vi "Find Turntable Centre.vi"(3 "Mode":T6=enum."Run VI", 5 "Traverse line In":T3={"Start X"=-1250.0, "Start Y"=-250.0, "Start Z"=180.0, "End X"=0.0, "End Y"=0.0, "End Z"=0.0, "No. of pts."=6, "Spacing"=enum."Linear", "Filename"=path "C:/Enflo_Data_Local/2015/EnFlo_Tunnel/Paul_Hayden/Calibrations/Cal_06-2015/Datum_Block_1.xls", "Tunnel Speed"=0.0, "Averaging time (min)"=0.01, "Extra Commands"="", "Carrier_1 Q (l/min)"=nan, "Carrier_2 Q (l/min)"=nan, "Trace Gas Concentration (%)"=nan, "Specific Arguments"="Datum_Image_Calibration.vi  ", "Comments"="", "Row No"=0, "Row Type Selector"=enum."Run VI Named:", "Completion time"="12:51  12-06-2015", "Row Duration (mins)"=0.11291999999999999, "No. of Valid pts."=6, "Meas Setup File"="Trav_Cam_Picture.xls"} {"Carrier_2 Q (l/min)" format="%#.2f"; "Row Duration (mins)" format="%#.1f"; "Row No" min=0; "Trace Gas Concentration (%)" min=0.0 format="%#_4f"; "Carrier_1 Q (l/min)" format="%#.2f"; "Tunnel Speed" format="%#.2f"; "Start X" format="%#.2f"; "Start Y" format="%#.2f"; "Start Z" format="%#.2f"; "End X" format="%#.2f"; "End Y" format="%#.2f"; "End Z" format="%#.2f"; "Averaging time (min)" min=0.0 format="%#.2f"}) -> (0 "Error Message":string, 1 "Status":T2, 2 "Traverse line Out":T3 {"Carrier_2 Q (l/min)" format="%#.2f"; "Row Duration (mins)" format="%#.1f"; "Row No" min=0; "Trace Gas Concentration (%)" min=0.0 format="%#_4f"; "Carrier_1 Q (l/min)" format="%#.2f"; "Tunnel Speed" format="%#.2f"; "Start X" format="%#.2f"; "Start Y" format="%#.2f"; "Start Z" format="%#.2f"; "End X" format="%#.2f"; "End Y" format="%#.2f"; "End Z" format="%#.2f"; "Averaging time (min)" min=0.0 format="%#.2f"})   [LabVIEW 2017]
uses:
  Gen Trav/Traverse_cluster.ctl
  Gen Trav/Spacing.ctl
  Controls/Multi_run_mode.ctl
  Controls/User_Specific_mode.ctl
  Gen Trav/Multi_Run_Status.ctl
  Camera Server/Camera enum/Camera enum.ctl
  Utilities/Image acquisition and processing/Feature detection/Typedefs/Top level controls.ctl
  Utilities/Image acquisition and processing/Feature detection/Typedefs/Theta range.ctl
  Utilities/Image acquisition and processing/Feature detection/Typedefs/Txy range.ctl
  Utilities/Image acquisition and processing/Feature detection/Typedefs/ROI bounds.ctl
  Camera Server/Camera enum/Camera resolution.ctl
  Controls/Setup.ctl
  Controls/Save_Data.ctl
  Globals/Constants_global.vi
  Globals/Dynamic_call_global.ph.vi
panel:
  out "Y Offset":dbl=-999.0 format="%.2f"
  out "X Offset":dbl=-999.0 format="%.2f"
  in  "Camera":T1="Travcam"
  out "Local Log File":path
  out "y radius":dbl
  out "x radius":dbl
  out "y centre 2":dbl
  out "x centre 2":dbl
  in  "stop":bool
  out "radius":dbl
  out "y centre":dbl
  out "x centre":dbl
  out "Y":dbl[](array[numeric])
  out "X":dbl[](array[numeric])
  in  "Radius":dbl=900.0
  # "Circle"
  # "Ellipse"
  # "X           Y            Z"
  # "Start"
  # "End"
  # "X           Y            Z"
  # "Start"
  # "End"
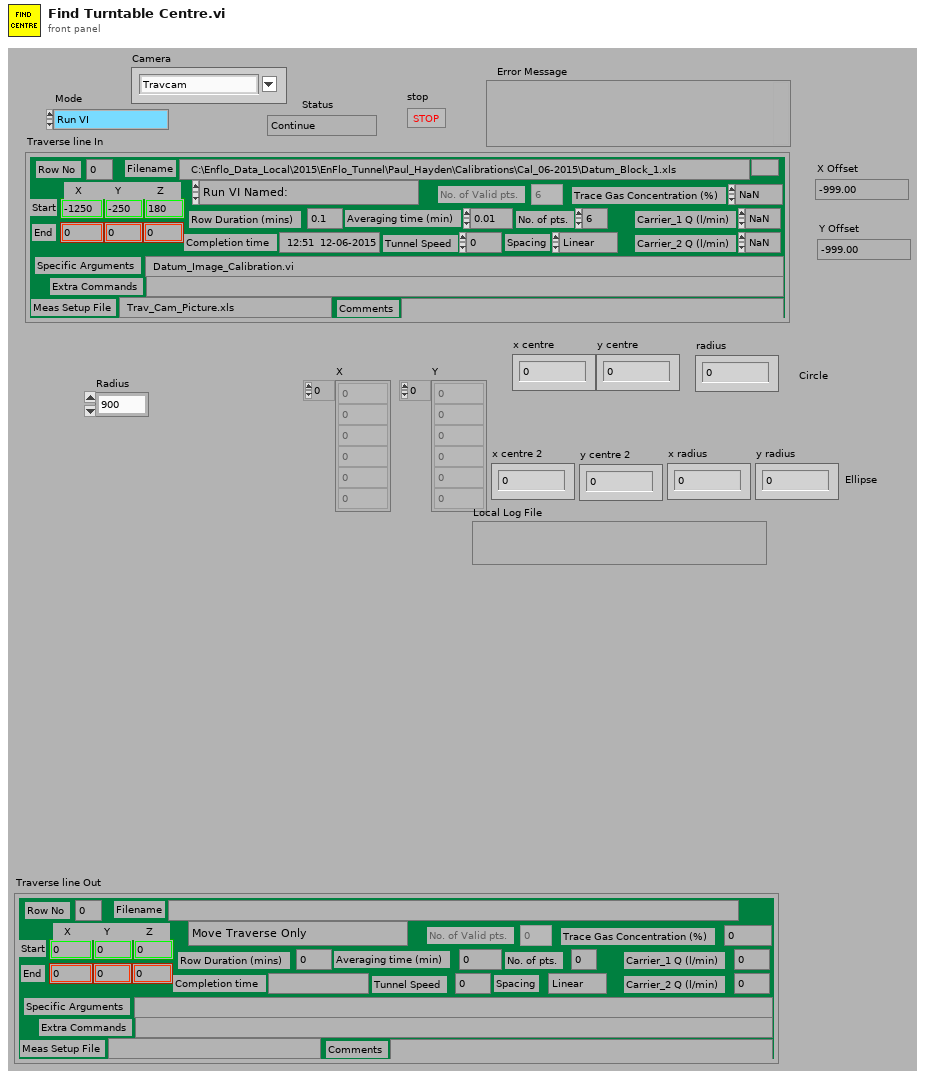
[diagram p1: front panel]
types:
  T1 = typedef "Camera enum.ctl" = string
  T2 = typedef "Multi_Run_Status.ctl" = enum16{"Continue", "Continue with Error", "Jump to Next Point", "Jump to Next Row", "Jump To Fall Back", "Terminate Run"}
  T3 = typedef "Traverse_cluster.ctl" = cluster{"Start X":sgl, "Start Y":sgl, "Start Z":sgl, "End X":sgl, "End Y":sgl, "End Z":sgl, "No. of pts.":i32, "Spacing":T4, "Filename":path, "Tunnel Speed":dbl, "Averaging time (min)":dbl, "Extra Commands":string, "Carrier_1 Q (l/min)":dbl, "Carrier_2 Q (l/min)":dbl, "Trace Gas Concentration (%)":dbl, "Specific Arguments":string, "Comments":string, "Row No":i32, "Row Type Selector":T5, "Completion time":string, "Row Duration (mins)":dbl, "No. of Valid pts.":i32, "Meas Setup File":string}
  T4 = typedef "Spacing.ctl" = enum16{"Linear", "Log", "Gauss", "Specified", "N/A"}
  T5 = typedef "Multi_run_mode.ctl" = enum16{"Move Traverse Only", "Set Tunnel Speed Only", "Set Source Only", "Set Measurement Conditions", "Single Measurement", "Vertical Profile", "Lateral Profile", "Longitudinal Profile", "Explore Volume", "Multi-Axis Profile", "Auto Calibrate", "Meas Fast FID Bkgnd", "Check Beam Power", "Scanning Valve Measurement", "Run VI Named:", "Set ADAM Ch", "Wait (minutes)", "Send Message", "Synchronize With:", "Fall Back to this Row", "Turn Off Row Repeating", "Traverse 3D Volume", "Blank Row", "Jump to Fall Back Row"}
  T6 = typedef "User_Specific_mode.ctl" = enum16{"Check VI only", "Run VI"}
  T7 = typedef "ROI bounds.ctl" = cluster{"Xmax":i32, "Ymax":i32, "Xmin":i32, "Ymin":i32}
  T8 = typedef "Txy range.ctl" = cluster{"Tx max (pix)":i32, "Tx min (pix)":i32, "Ty max (pix)":i32, "Ty min (pix)":i32}
  T9 = typedef "Theta range.ctl" = cluster{"theta max (deg)":dbl, "theta min (deg)":dbl}
  T10 = typedef "Top level controls.ctl" = cluster{"Auto ROI (for rot.)":bool, "Apply scaling":bool, "Apply rotation":bool, "Apply Tx":bool, "Apply Ty":bool, "Keep proc. img":bool}
  T11 = typedef "Save_Data.ctl" = enum16{"Save No Data", "Save Data"}
  T12 = typedef "Setup.ctl" = enum16{"Run Program", "Show Setup", "Save Current Setup", "Setup Front Panel"}
  T13 = typedef "Camera resolution.ctl" = u8
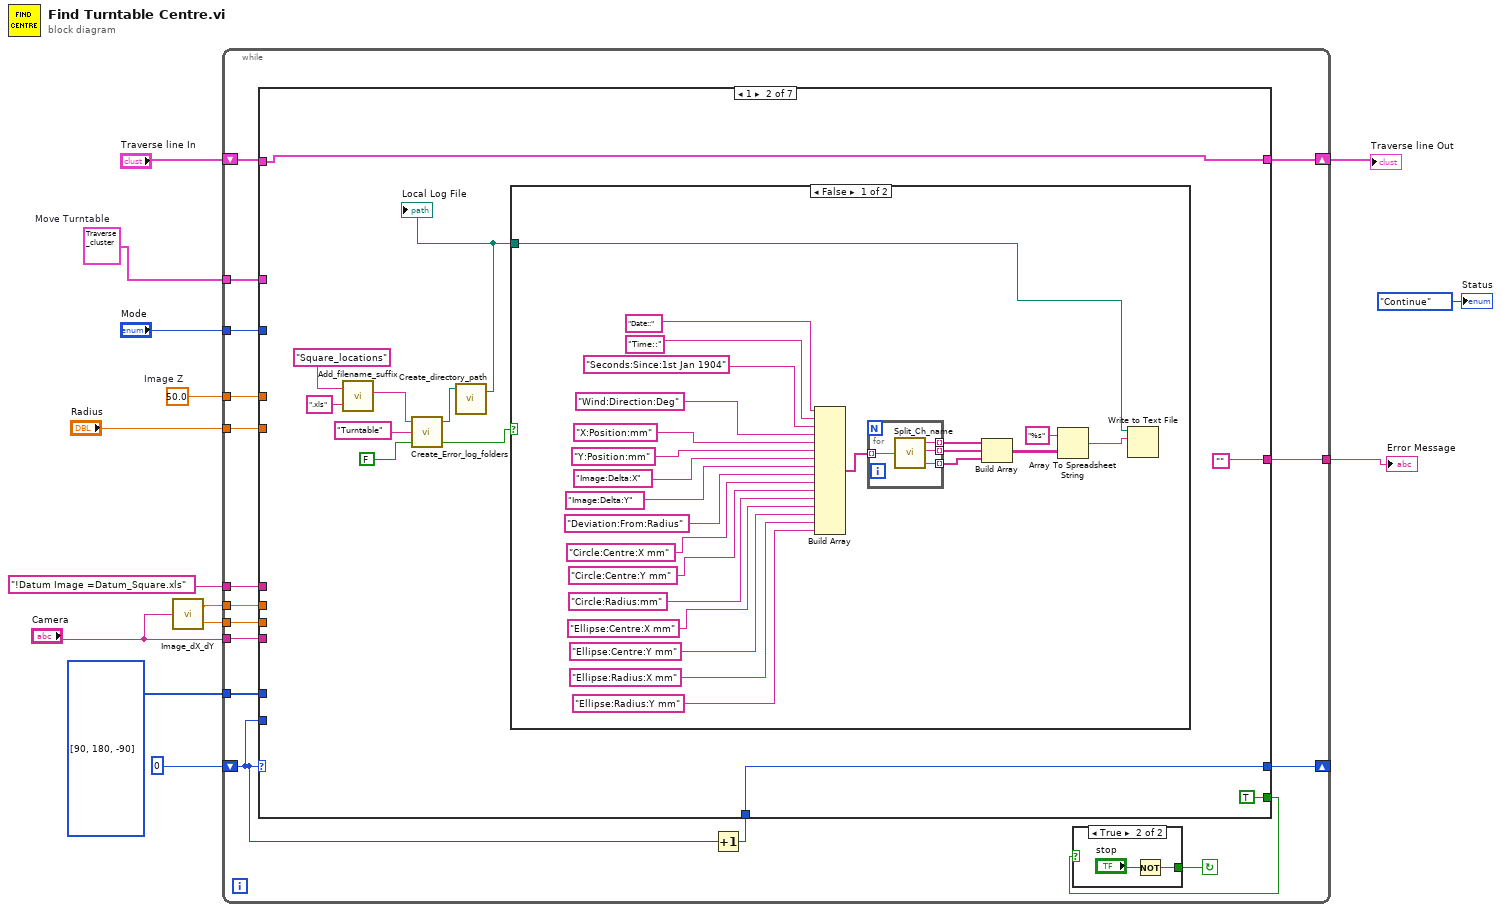
[diagram p0: block diagram]
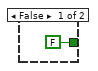
[diagram p2: hidden frame]
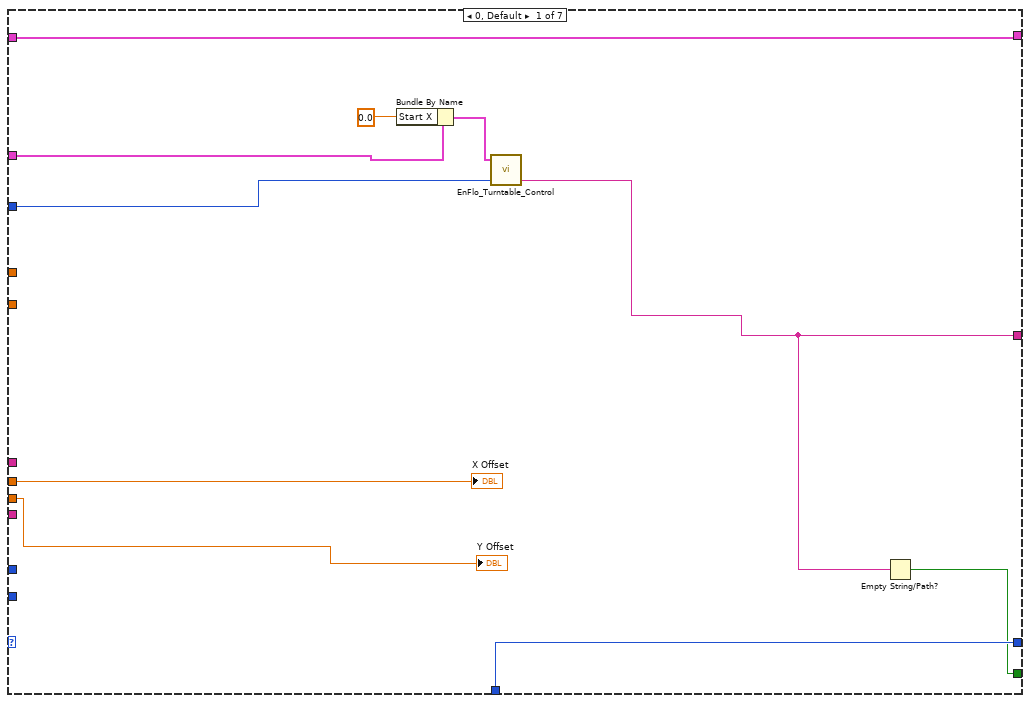
[diagram p3: hidden frame]
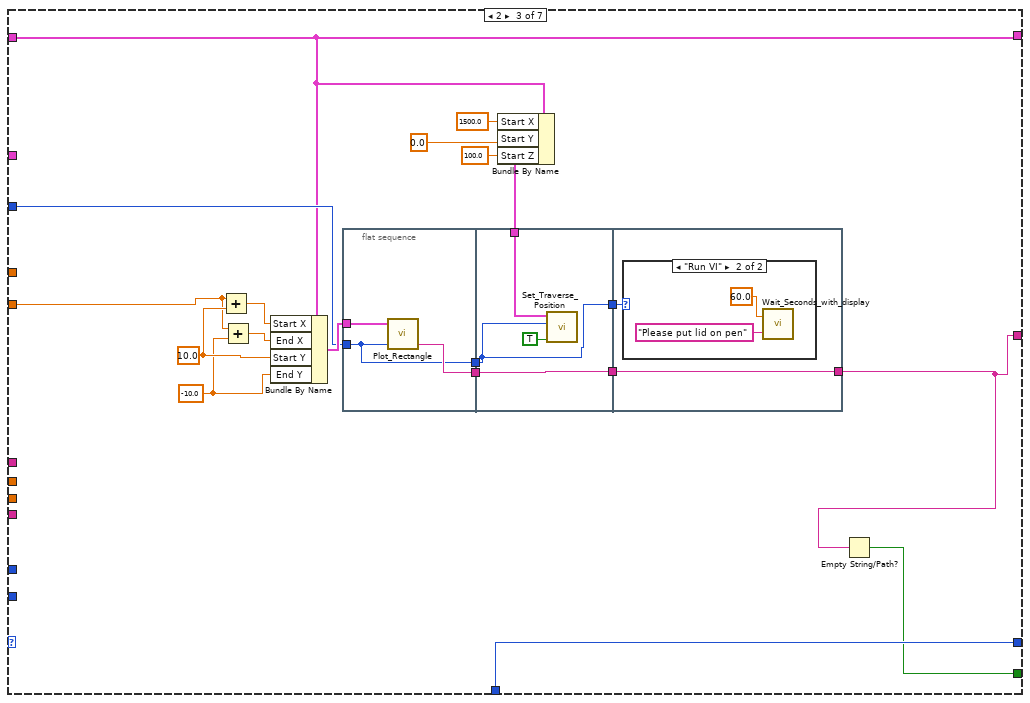
[diagram p5: hidden frame]
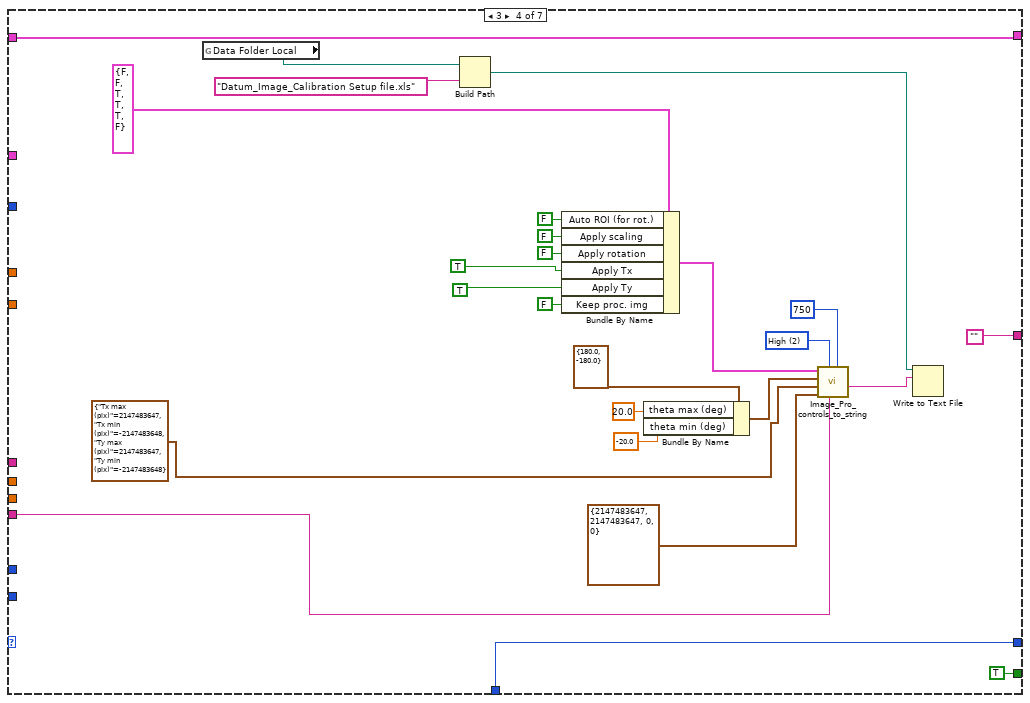
[diagram p7: hidden frame]
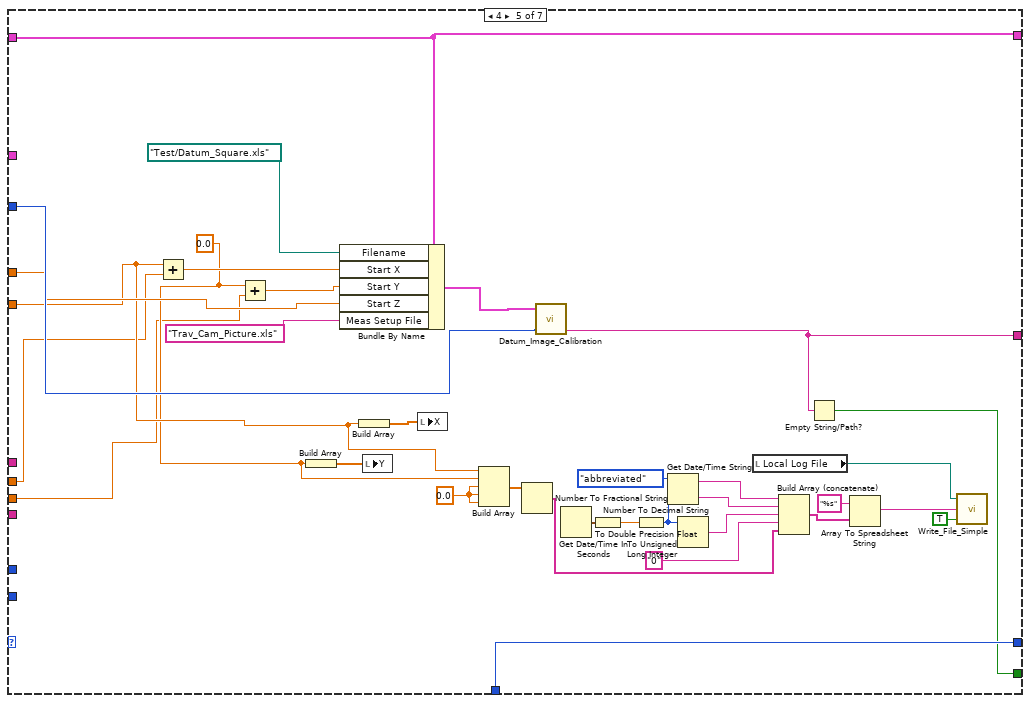
[diagram p8: hidden frame]
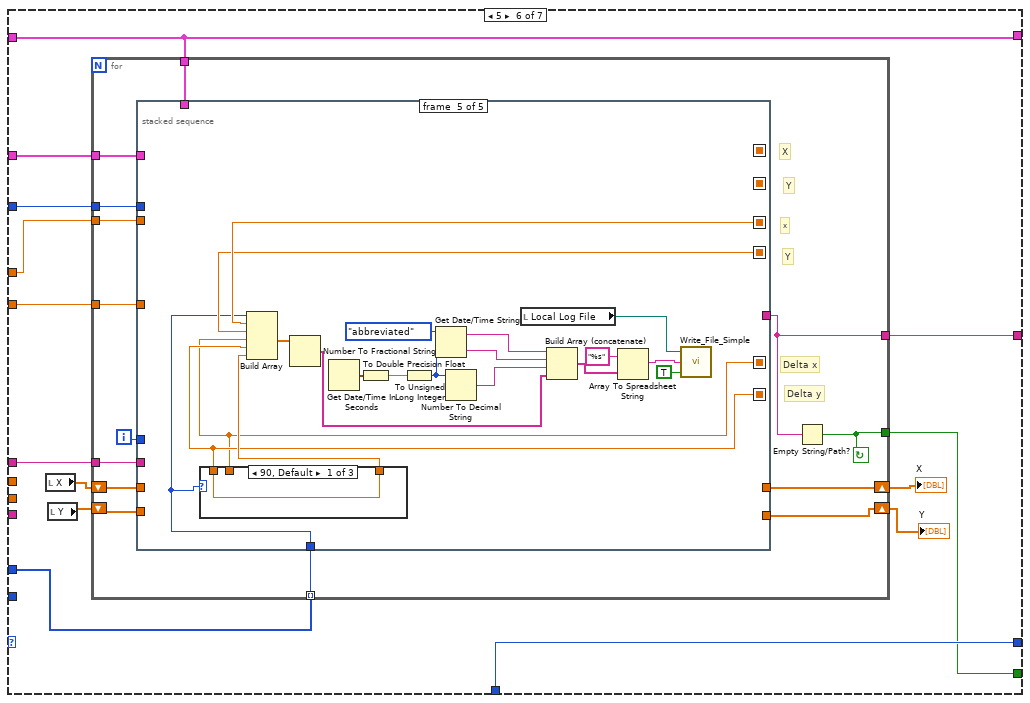
[diagram p9: hidden frame]
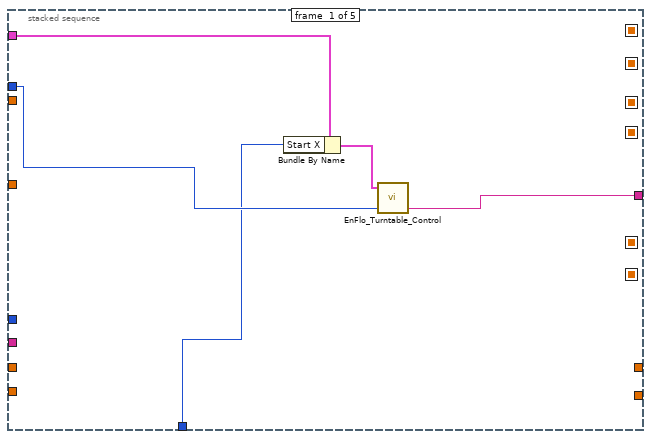
[diagram p10: hidden frame]
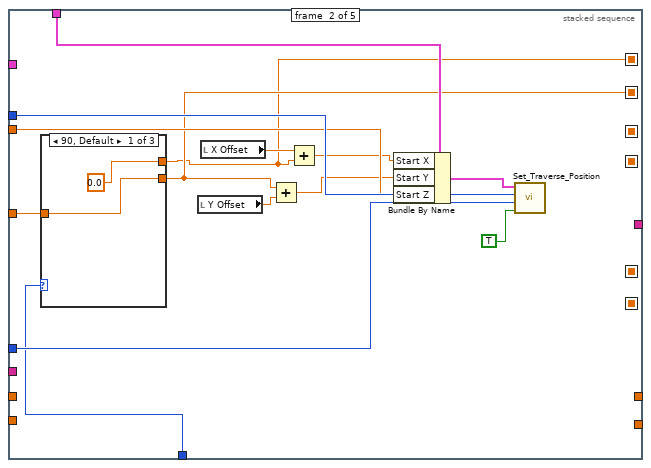
[diagram p11: hidden frame]
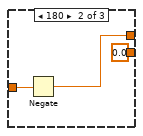
[diagram p12: hidden frame]
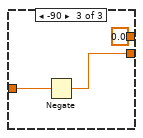
[diagram p13: hidden frame]
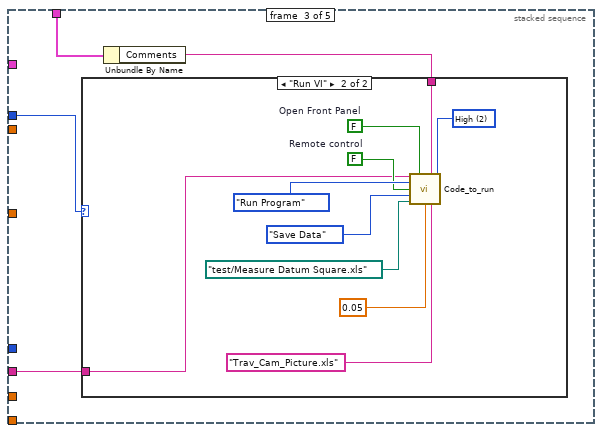
[diagram p14: hidden frame]
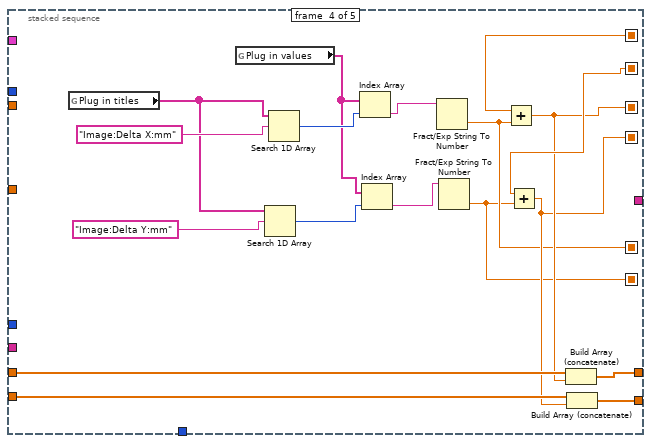
[diagram p16: hidden frame]
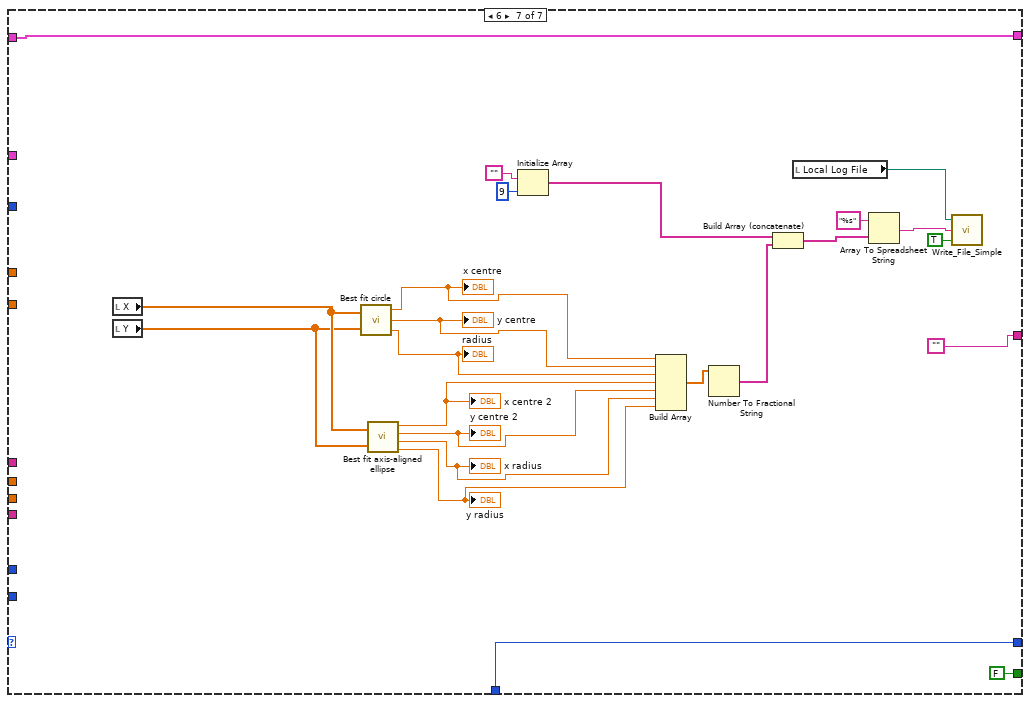
[diagram p19: hidden frame]
diagram:
  w4 = T3 {"Start X"=0.0, "Start Y"=nan, "Start Z"=nan, "End X"=nan, "End Y"=nan, "End Z"=nan, "No. of pts."=0, "Spacing"=enum."N/A", "Filename"=path "  ---------", "Tunnel Speed"=nan, "Averaging time (min)"=nan, "Extra Commands"="!Datum Image = Datum_Turntable.xls", "Carrier_1 Q (l/min)"=nan, "Carrier_2 Q (l/min)"=nan, "Trace Gas Concentration (%)"=nan, "Specific Arguments"="EnFlo_Turntable_Control.vi", "Comments"="", "Row No"=0, "Row Type Selector"=enum."Run VI Named:", "Completion time"="18:36  07-04-2016", "Row Duration (mins)"=0.6666666666666666, "No. of Valid pts."=0, "Meas Setup File"="Trav_Cam_Picture.xls"}  # Move Turntable
  w7 = sgl 50.0  # Image Z
  n1 = call "Image_dX_dY.vi"("Camera"="Camera") -> ("X Offset"=w2:dbl, "Y Offset"=w1:dbl)
  n2 = while {
    shift-left: 0 -> [w27]
    shift-right: [w31] -> _
    tunnel: "Mode" -> [w30]
    shift-right: [w28] -> w11
    shift-left: "Traverse line In" -> [w29]
    tunnel: "Radius" -> [w25]
    tunnel: [w24] -> w9
    tunnel: w7 -> [w23]
    tunnel: i32[] [90, 180, -90] ("appended array") -> [w20]
    tunnel: "!Datum Image =Datum_Square.xls" ("Extra Commands") -> [w19]
    tunnel: w4 -> [w18]
    tunnel: "Camera" -> [w17]
    tunnel: w2 -> [w16]
    tunnel: w1 -> [w15]
    stop <- w21 continue-if-true
    n3 = Increment(x=w27) -> (x+1=w26:i32)
    n4 = case shown="1" w27 {
      tunnel: [w42 TRUE w100 TRUE w168 w183 FALSE] -> w22
      tunnel: [w44 w49 w102 w139 w171 w186 w302] -> w31
      tunnel: w27 -> [_ _ _ _ _ _ _]
      tunnel: w30 -> [w41 _ w101 _ w166 w185 _]
      tunnel: w29 -> [w43 w50 w93 w138 w172 w181 w303]
      tunnel: [w43 w50 w93 w138 w172 w181 w303] -> w28
      tunnel: w26 -> [w44 w49 w102 w139 w171 w186 w302]
      tunnel: w25 -> [_ _ w96 _ w147 w182 _]
      tunnel: [w38 "" w86 "" w165 w184 ""] -> w24
      tunnel: w23 -> [_ _ _ _ w162 w176 _]
      tunnel: w20 -> [_ _ _ _ _ w175 _]
      tunnel: w19 -> [_ _ _ _ _ w174 _]
      tunnel: w18 -> [w37 _ _ _ _ w173 _]
      tunnel: w17 -> [_ _ _ w117 _ _ _]
      tunnel: w16 -> [w36 _ _ _ w144 _ _]
      tunnel: w15 -> [w35 _ _ _ w143 _ _]
      frame 0, Default {
        n5 = Bundle By Name(cluster=w37, "Start X"=sgl 0.0 ("element")) -> (w40:T3)
        n6 = call "EnFlo_Turntable_Control.vi"("Mode"=w41, "Traverse line In"=w40) -> ("Error Message"=w38:string)  [unwired: 1 in, 2 out]
        n7 = Empty String/Path?(string/path=w38) -> (empty?=w42:bool)
        "X Offset" <- w36
        "Y Offset" <- w35
      }
      frame 1 {
        n8 = call "Add_filename_suffix.vi"("Filename"="Square_locations", "Suffix to add"=".xls") -> ("Filename out"=w54:string)  [unwired: 3 out]
        n9 = call "Create_Error_log_folders.vi"("Log Filename"=w54, "Log Folder"="Turntable" ("Input Element"), "Per Day Log File?"=FALSE) -> ("Local Log File"=w46:path, "exists?"=w52:bool)  [unwired: 2 in, 1 out]
        n10 = call "Create_directory_path.vi"("Path name"=w46) -> ("Path name Out"=w45:path)  [unwired: 2 in, 1 out]
        "Local Log File" <- w45
        n11 = case shown="False" w52 {
          tunnel: w45 -> [w67 _]
          frame False {
            n12 = Build Array("Date::", "Time::", "Seconds:Since:1st Jan 1904", "Wind:Direction:Deg", "X:Position:mm", "Y:Position:mm", "Image:Delta:X", "Image:Delta:Y", "Deviation:From:Radius", "Circle:Centre:X mm", "Circle:Centre:Y mm", "Circle:Radius:mm", "Ellipse:Centre:X mm", "Ellipse:Centre:Y mm", "Ellipse:Radius:X mm", "Ellipse:Radius:Y mm") -> (w76:string[])
            n13 = for {
              tunnel: w76 -> [w84] mode=indexing
              tunnel: [w83] -> w75 mode=indexing
              tunnel: [w82] -> w74 mode=indexing
              tunnel: [w81] -> w73 mode=indexing
              n14 = call "Split_Ch_name.vi"("Ch name"=w84) -> ("Top level"=w83:string, "Middle"=w82:string, "Low level"=w81:string)
            }
            n15 = Build Array(w75, w74, w73) -> (w65:string[][])
            n16 = Array To Spreadsheet String(array=w65, 3:"%s" ("format string")) -> (spreadsheet string=w64:string)  [unwired: 1 out]
            n17 = Write to Text File(file (use dialog)=w67, text=w64) -> ()  [unwired: 2 in, 3 out]
          }
          frame True {
          }
        }
      }
      frame 2 {
        w97 = sgl -10.0 ("End Y")
        w98 = sgl 10.0 ("Start Y")
        n18 = Add(x=w96, y=w98) -> (x+y=w99:dbl)
        n19 = Add(x=w96, y=w97) -> (x+y=w95:dbl)
        n20 = Bundle By Name(cluster=w93, "Start X"=w99, "End X"=w95, "Start Y"=w98, "End Y"=w97) -> (w103:T3)
        n21 = flat-sequence {
          tunnel: [w105] -> w94
          tunnel: [w104] -> w88
          tunnel: w103 -> [w106]
          tunnel: w101 -> [w104]
          tunnel: w94 -> [w110]
          tunnel: w89 -> [w109]
          tunnel: w88 -> [w107]
          tunnel: [w110] -> w87
          tunnel: [w107] -> w85
          tunnel: [w112] -> w86
          tunnel: w87 -> [w112]
          tunnel: w85 -> [w111]
          frame #0 {
            n22 = call "Plot_Rectangle.vi"("Mode"=w104, "Traverse line In"=w106) -> ("Error Message"=w105:string)  [unwired: 1 in, 2 out]
          }
          frame #1 {
            n23 = call "Set_Traverse_Position.vi"("Last Part of Move?"=TRUE, "Simulate/Run"=w107, "Traverse line"=w109) -> ()  [unwired: 3 in, 1 out]
          }
          frame #2 {
            n24 = case shown="\"Run VI\"" w111 {
              frame "Check VI only" {
              }
              frame "Run VI" {
                n25 = call "Wait_Seconds_with_display.vi"("Message"="Please put lid on pen", "Seconds to wait"=60.0) -> ()  [unwired: 1 in, 1 out]
              }
            }
          }
        }
        n26 = Bundle By Name(cluster=w93, "Start X"=sgl 1500.0, "Start Y"=sgl 0.0, "Start Z"=sgl 100.0) -> (w89:T3)
        n27 = Empty String/Path?(string/path=w86) -> (empty?=w100:bool)
      }
      frame 3 {
        w116 = T13 2 items=["Low", "Med.", "High", "Max."] ("Resolution")
        n28 = global read "Constants_global.vi" "Data Folder Local"() -> (w136:path)
        n29 = Build Path(base path=w136, name or relative path="Datum_Image_Calibration Setup file.xls") -> (appended path=w121:path)
        n30 = Bundle By Name(cluster=T10 {"Auto ROI (for rot.)"=FALSE, "Apply scaling"=FALSE, "Apply rotation"=TRUE, "Apply Tx"=TRUE, "Apply Ty"=TRUE, "Keep proc. img"=FALSE} ("Controls"), "Auto ROI (for rot.)"=FALSE, "Apply scaling"=FALSE, "Apply rotation"=FALSE, "Apply Tx"=TRUE, "Apply Ty"=TRUE, "Keep proc. img"=FALSE) -> (w128:T10)
        n31 = Bundle By Name(cluster=T9 {"theta max (deg)"=180.0, "theta min (deg)"=-180.0} ("Theta range (deg)"), "theta max (deg)"=20.0, "theta min (deg)"=-20.0) -> (w126:T9)
        n32 = call "Image_Pro_controls_to_string.vi"("Quality"=u32 750, "Camera"=w117, "Resolution"=w116, "ROI to crop (pixels)"=T7 {"Xmax"=2147483647, "Ymax"=2147483647, "Xmin"=0, "Ymin"=0}, "Txy range (pixels)"=T8 {"Tx max (pix)"=2147483647, "Tx min (pix)"=-2147483648, "Ty max (pix)"=2147483647, "Ty min (pix)"=-2147483648}, "Theta range (deg)"=w126, "Controls"=w128) -> ("Setup String"=w122:string)  [unwired: 4 in]
        n33 = Write to Text File(file (use dialog)=w121, text=w122) -> ()  [unwired: 2 in, 3 out]
      }
      frame 4 {
        w152 = 0.0 ("element")
        w146 = sgl 0.0 ("Start Y")
        n34 = Add(x=w147, y=w144) -> (x+y=w153:dbl)
        n35 = Add(x=w146, y=w143) -> (x+y=w145:dbl)
        n36 = Build Array(w146) -> (w163:sgl[])
        n37 = Bundle By Name(cluster=w172, "Filename"=path "Test/Datum_Square.xls", "Start X"=w153, "Start Y"=w145, "Start Z"=w162, "Meas Setup File"="Trav_Cam_Picture.xls") -> (w167:T3)
        n38 = Build Array(w147) -> (w164:dbl[])
        n39 = local write "Y"(w163) -> ()
        n40 = local write "X"(w164) -> ()
        n41 = Build Array(w147, w146, w152, w152, w152) -> (w151:dbl[])
        n42 = Number To Fractional String(number=w151) -> (F-format string=w150:string[])  [unwired: 3 in]
        n43 = call "Datum_Image_Calibration.vi"("Mode"=w166, "Traverse line In"=w167) -> ("Error Message"=w165:string)  [unwired: 1 in, 2 out]
        n44 = Get Date/Time In Seconds() -> (seconds since 1Jan1904=w158:timestamp)
        n45 = To Double Precision Float(number=w158) -> (double precision float=w160:dbl)
        n46 = To Unsigned Long Integer(number=w160) -> (unsigned 32bit integer=w159:u32)
        n47 = Get Date/Time String(date format (0)=enum16{"short", "long", "abbreviated"}."abbreviated", seconds (now)=w159) -> (date string=w157:string, time string=w156:string)  [unwired: 1 out]
        n48 = Number To Decimal String(number=w159) -> (decimal integer string=w155:string)  [unwired: 1 out]
        n49 = local read "Local Log File"() -> (w142:path)
        n50 = Build Array (concatenate)(w157, w156, w155, "0", w150) -> (w148:string[])
        n51 = Empty String/Path?(string/path=w165) -> (empty?=w168:bool)
        n52 = Array To Spreadsheet String(array=w148, 3:"%s" ("format string")) -> (spreadsheet string=w141:string)  [unwired: 1 out]
        n53 = call "Write_File_Simple.vi"("append to file? (new file:F)"=TRUE, "character string"=w141, "file path"=w142) -> ()  [unwired: 2 out]
      }
      frame 5 {
        n54 = local read "X"() -> (w180:dbl[])
        n55 = local read "Y"() -> (w179:dbl[])
        n56 = for {
          tunnel: w185 -> [w200]
          tunnel: [w199] -> w184
          tunnel: [w198] -> w183
          tunnel: w175 -> [w197] mode=indexing
          tunnel: w182 -> [w196]
          tunnel: w181 -> [w195]
          shift-right: [w191] -> w178
          shift-left: w180 -> [w193]
          shift-right: [w190] -> w177
          shift-left: w179 -> [w192]
          tunnel: w176 -> [w189]
          tunnel: w174 -> [w188]
          tunnel: w173 -> [w187]
          i -> [w194]
          stop <- w198 continue-if-true
          # "Y"
          # "X"
          # "Delta y"
          # "Delta x"
          # "Y"
          # "x"
          n57 = stacked-sequence {
            seq-local: [_ w206 _ _ _] -> [_ _ _ w251 _]
            seq-local: [_ w209 _ _ _] -> [_ _ _ w250 _]
            seq-local: [_ _ _ w245 _] -> [_ _ _ _ w268]
            seq-local: [_ _ _ w244 _] -> [_ _ _ _ w267]
            seq-local: [_ _ _ w243 _] -> [_ _ _ _ w263]
            seq-local: [_ _ _ w242 _] -> [_ _ _ _ w264]
            tunnel: w200 -> [w204 w218 w231 _ _]
            tunnel: [w201 _ _ _ _] -> w199
            tunnel: w197 -> [w203 w212 _ _ w266]
            tunnel: w196 -> [_ w215 _ _ _]
            tunnel: w195 -> [_ w219 w229 _ _]
            tunnel: w194 -> [_ w216 _ _ _]
            tunnel: w193 -> [_ _ _ w249 _]
            tunnel: w192 -> [_ _ _ w248 _]
            tunnel: [_ _ _ w247 _] -> w191
            tunnel: [_ _ _ w246 _] -> w190
            tunnel: w189 -> [_ w213 _ _ _]
            tunnel: w188 -> [_ _ w230 _ _]
            tunnel: w187 -> [w202 _ _ _ _]
            frame #0 {
              n58 = Bundle By Name(cluster=w202, "Start X"=w203) -> (w205:T3)
              n59 = call "EnFlo_Turntable_Control.vi"("Mode"=w204, "Traverse line In"=w205) -> ("Error Message"=w201:string)  [unwired: 1 in, 2 out]
            }
            frame #1 {
              n60 = case shown="90, Default" w212 {
                tunnel: [0.0 ("X Offset from Camera") w222 0.0 ("X Offset from Camera")] -> w206
                tunnel: w215 -> [w221 w223 w227]
                tunnel: [w221 0.0 ("X position") w226] -> w209
                frame 90, Default {
                }
                frame 180 {
                  n61 = Negate(x=w223) -> (-x=w222:dbl)
                }
                frame -90 {
                  n62 = Negate(x=w227) -> (-x=w226:dbl)
                }
              }
              n63 = local read "Y Offset"() -> (w210:dbl)
              n64 = local read "X Offset"() -> (w207:dbl)
              n65 = Add(x=w209, y=w210) -> (x+y=w208:dbl)
              n66 = Add(x=w207, y=w206) -> (x+y=w211:dbl)
              n67 = Bundle By Name(cluster=w219, "Start X"=w211, "Start Y"=w208, "Start Z"=w213) -> (w214:T3)
              n68 = call "Set_Traverse_Position.vi"("Last Part of Move?"=TRUE, "Currently on Point"=w216, "Simulate/Run"=w218, "Traverse line"=w214) -> ()  [unwired: 2 in, 1 out]
            }
            frame #2 {
              n69 = Unbundle By Name(w229) -> ("Comments"=w228:string)
              n70 = case shown="\"Run VI\"" w231 {
                tunnel: w230 -> [_ w234]
                tunnel: w228 -> [_ w233]
                frame "Check VI only" {
                }
                frame "Run VI" {
                  w232 = T13 2 items=["Low", "Med.", "High", "Max."] ("Camera Resolution")
                  w239 = FALSE  # Open Front Panel
                  w238 = FALSE  # Remote control
                  n71 = call "Code_to_run.vi"("Extra command String"=w234, "Open Front Panel"=w239, "Current Row Comments"=w233, "Camera Resolution"=w232, "setup"=Setup."Run Program", "Remote control"=w238, "File"=Save_Data."Save Data", "Results Filename"=path "test/Measure Datum Square.xls", "Averaging time (min)"=0.05, "Setup filename"="Trav_Cam_Picture.xls" ("Extra Commands")) -> ()  [unwired: 2 in, 4 out]
                }
              }
            }
            frame #3 {
              n72 = global read "Dynamic_call_global.ph.vi" "Plug in titles"() -> (w255:string[])
              n73 = global read "Dynamic_call_global.ph.vi" "Plug in values"() -> (w254:string[])
              n74 = Search 1D Array(1D array=w255, element="Image:Delta Y:mm") -> (index of element=w253:i32)  [unwired: 1 in]
              n75 = Search 1D Array(1D array=w255, element="Image:Delta X:mm") -> (index of element=w258:i32)  [unwired: 1 in]
              n76 = Index Array(array=w254, index=w258) -> (element=w259:string)
              n77 = Index Array(array=w254, index=w253) -> (element=w252:string)
              n78 = Fract/Exp String To Number(string=w259) -> (number=w243:dbl)  [unwired: 3 in, 1 out]
              n79 = Fract/Exp String To Number(string=w252) -> (number=w242:dbl)  [unwired: 3 in, 1 out]
              n80 = Add(x=w251, y=w243) -> (x+y=w245:dbl)
              n81 = Add(x=w250, y=w242) -> (x+y=w244:dbl)
              n82 = Build Array (concatenate)(w249, w245) -> (w247:dbl[])
              n83 = Build Array (concatenate)(w248, w244) -> (w246:dbl[])
            }
            frame #4 {
              n84 = case shown="90, Default" w266 {
                tunnel: [w280 w281 w282] -> w265
                tunnel: w264 -> [w280 w281 _]
                tunnel: w263 -> [_ _ w282]
                frame 90, Default {
                }
                frame -90 {
                }
                frame 180 {
                }
              }
              n85 = Build Array(w266, w268, w267, w263, w264, w265) -> (w272:dbl[])
              n86 = Number To Fractional String(number=w272) -> (F-format string=w271:string[])  [unwired: 3 in]
              n87 = Get Date/Time In Seconds() -> (seconds since 1Jan1904=w276:timestamp)
              n88 = To Double Precision Float(number=w276) -> (double precision float=w278:dbl)
              n89 = To Unsigned Long Integer(number=w278) -> (unsigned 32bit integer=w277:u32)
              n90 = Get Date/Time String(date format (0)=enum16{"short", "long", "abbreviated"}."abbreviated", seconds (now)=w277) -> (date string=w275:string, time string=w274:string)  [unwired: 1 out]
              n91 = Number To Decimal String(number=w277) -> (decimal integer string=w273:string)  [unwired: 1 out]
              n92 = local read "Local Log File"() -> (w260:path)
              n93 = Build Array (concatenate)(w275, w274, w273, w271) -> (w269:string[])
              n94 = Array To Spreadsheet String(array=w269, 3:"%s" ("format string")) -> (spreadsheet string=w261:string)  [unwired: 1 out]
              n95 = call "Write_File_Simple.vi"("append to file? (new file:F)"=TRUE, "character string"=w261, "file path"=w260) -> ()  [unwired: 2 out]
            }
          }
          n96 = Empty String/Path?(string/path=w199) -> (empty?=w198:bool)
        }
        "X" <- w178
        "Y" <- w177
      }
      frame 6 {
        n97 = local read "X"() -> (w301:dbl[])
        n98 = local read "Y"() -> (w300:dbl[])
        n99 = call "Best fit circle.vi"("x array"=w301, "y array"=w300) -> ("x centre"=w294:dbl, "y centre"=w293:dbl, "radius"=w292:dbl)
        "x centre" <- w294
        "y centre" <- w293
        "radius" <- w292
        n100 = call "Best fit axis-aligned ellipse.vi"("x array"=w301, "y array"=w300) -> ("x centre"=w291:dbl, "y centre"=w290:dbl, "x radius"=w289:dbl, "y radius"=w288:dbl)
        "x centre 2" <- w291
        "y centre 2" <- w290
        "x radius" <- w289
        "y radius" <- w288
        n101 = Initialize Array("", 9 ("dimension size")) -> (w286:string[])
        n102 = Build Array(w294, w293, w292, w291, w290, w289, w288) -> (w287:dbl[])
        n103 = Number To Fractional String(number=w287) -> (F-format string=w299:string[])  [unwired: 3 in]
        n104 = Build Array (concatenate)(w286, w299) -> (w297:string[])
        n105 = local read "Local Log File"() -> (w283:path)
        n106 = Array To Spreadsheet String(array=w297, 3:"%s" ("format string")) -> (spreadsheet string=w284:string)  [unwired: 1 out]
        n107 = call "Write_File_Simple.vi"("append to file? (new file:F)"=TRUE, "character string"=w284, "file path"=w283) -> ()  [unwired: 2 out]
      }
    }
    n108 = case shown="True" w22 {
      tunnel: [FALSE ("stop") w33] -> w21
      frame False {
      }
      frame True {
        n109 = Not(x="stop") -> (.not. x?=w33:bool)
      }
    }
  }
  "Traverse line Out" <- w11
  "Error Message" <- w9
  "Status" <- Multi_Run_Status."Continue" ("Status")
